vi "initialize Session Data.vi"(0 "OBJ - Session in":refnum<class "Serial Session.lvclass">, 11 "error in":errorcluster) -> (4 "OBJ - Session out":refnum<class "Serial Session.lvclass">, 15 "error out":errorcluster)   [LabVIEW 2014, in "Serial Session.lvclass"]
doc: "OVERRIDE VI\nPlaceholder for decendant sessions to initialize and set their default values"
uses:
  Serial Session.lvclass
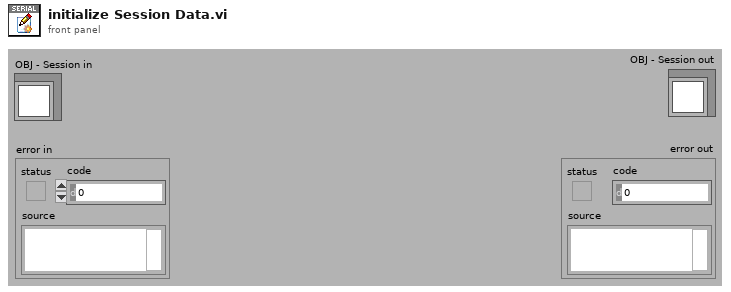
[diagram p1: front panel]
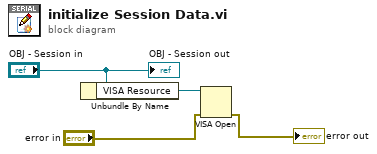
[diagram p0: block diagram]
diagram:
  n1 = Unbundle By Name("OBJ - Session in") -> ("VISA Resource"=w3:refnum<visa-resource-name>)
  n2 = VISA Open(error in (no error)="error in", VISA resource name=w3) -> (error out=→"error out":errorcluster)  [unwired: 3 in, 1 out]
  "OBJ - Session out" <- "OBJ - Session in"
